vi "SaveLibraryArray.vi"(6 "Total Project Progress":dbl, 7 "Project":refnum<vi>, 8 "error in (no error)":errorcluster, 11 "Library References":refnum<vi>[](array[refnum])) -> (0 "error out":errorcluster)   [LabVIEW 2016, in "NI_NPW_Project Copying.lvlib"]
uses:
  <resource>/dialog/NewProjectWizard/Project Copying/NI_NPW_Project Copying.lvlib
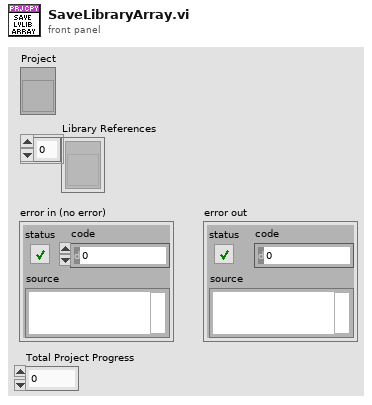
[diagram p1: front panel]
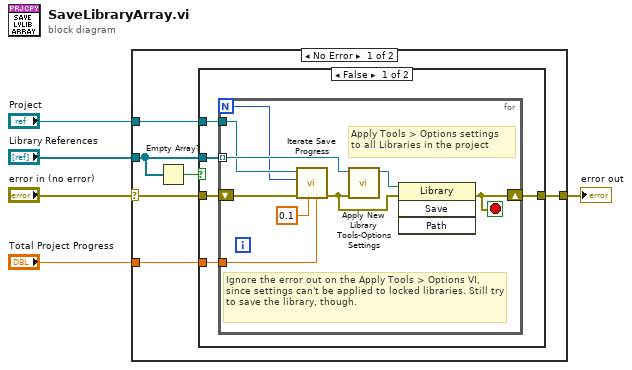
[diagram p0: block diagram]
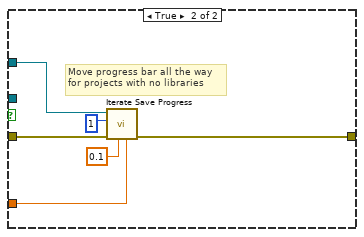
[diagram p2: hidden frame]
diagram:
  n1 = case shown="No Error" "error in (no error)" {
    selector: "error in (no error)" -> [w10 w32]
    tunnel: [w11 w32] -> w5
    tunnel: "Library References" -> [w7 _]
    tunnel: "Project" -> [w9 _]
    tunnel: "Total Project Progress" -> [w8 _]
    frame No Error {
      n2 = Empty Array?(array=w7) -> (empty?=w6:bool)
      n3 = case shown="False" w6 {
        tunnel: [w16 w27] -> w11
        tunnel: w10 -> [w15 w31]
        tunnel: w9 -> [w14 w30]
        tunnel: w8 -> [w13 w29]
        tunnel: w7 -> [w12 _]
        frame False {
          n4 = for {
            N -> [w18]
            tunnel: w12 -> [w25] mode=indexing
            shift-right: [w23] -> w16
            shift-left: w15 -> [w22]
            tunnel: w14 -> [w21]
            tunnel: w13 -> [w20]
            stop <- w23 stop-if-true
            # "Ignore the error out on the Apply Tools > Options VI, since settings can't be applied to locked libraries. Still try to save the library, though."
            # "Apply Tools > Options settings\nto all Libraries in the project"
            n5 = call <resource>:"Iterate Save Progress.vi"("Total Iteration Progress"=w20, "This Task's Percentage"=0.1, "error in (no error)"=w22, "Total Iterations (this task)"=w18, "Project"=w21) -> ("error out"=w17:errorcluster)  [unwired: 6 in]
            n6 = call <vilib>:"Apply New Library Tools-Options Settings.vi"("error in (no error)"=w17, "Library Refnum"=w25) -> ("dup Library Refnum"=w24:refnum<vi>)  [unwired: 8 in, 1 out]
            n7 = invoke class="Library" method="Save"(reference=w24, error in=w17) -> (error out=w23:errorcluster)  [unwired: 2 in, 3 out]
          }
        }
        frame True {
          # "Move progress bar all the way\nfor projects with no libraries"
          n8 = call <resource>:"Iterate Save Progress.vi"("Total Iteration Progress"=w29, "This Task's Percentage"=0.1, "error in (no error)"=w31, "Total Iterations (this task)"=1, "Project"=w30) -> ("error out"=w27:errorcluster)  [unwired: 6 in]
        }
      }
    }
    frame Error {
    }
  }
  "error out" <- w5
